vi "Mediaplayer play.vi"(0 "music":string(combo)="0", 2 "MediaPlayer":refnum<k7>(container), 3 "error in":errorcluster) -> (7 "error out":errorcluster)   [LabVIEW 2010]
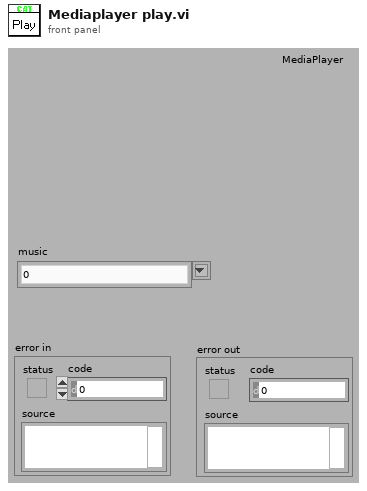
[diagram p1: front panel]
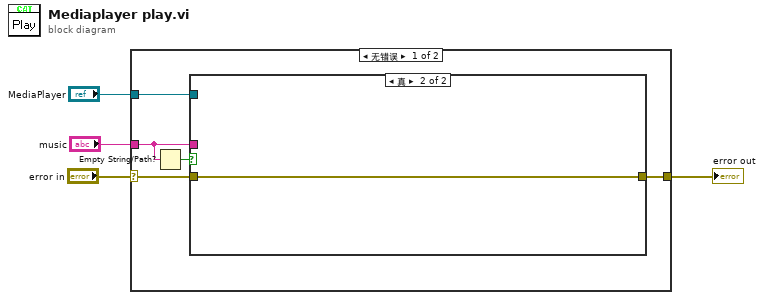
[diagram p0: block diagram]
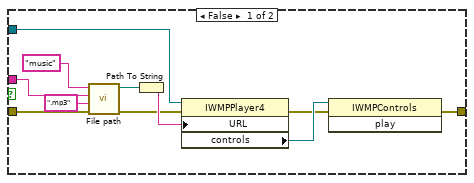
[diagram p2: hidden frame]
diagram:
  n1 = case shown="无错误" "error in" {
    selector: "error in" -> [w7 w22]
    tunnel: "music" -> [w5 _]
    tunnel: [w8 w22] -> w3
    tunnel: "MediaPlayer" -> [w9 _]
    frame No Error {
      n2 = Empty String/Path?(string/path=w5) -> (empty?=w6:bool)
      n3 = case shown="真" w6 {
        tunnel: w5 -> [w19 _]
        tunnel: w9 -> [w16 _]
        tunnel: [w13 w21] -> w8
        tunnel: w7 -> [w12 w21]
        frame False {
          n4 = call "File path.vi"("folder name"="music", "file name"=w19, "pattern"=".mp3", "error in (no error)"=w12) -> ("build path"=w11:path, "error out"=w17:errorcluster)  [unwired: 3 out]
          n5 = Path To String(path=w11) -> (string=w18:string)
          n6 = property class="IWMPPlayer4"(reference=w16, error in=w17, "URL"=w18) -> (error out=w14:errorcluster, "controls"=w15:refnum<k7>)  [unwired: 1 out]
          n7 = invoke class="IWMPControls" method="play"(reference=w15, error in=w14) -> (error out=w13:errorcluster)  [unwired: 1 in, 2 out]
        }
        frame True {
        }
      }
    }
    frame Error {
    }
  }
  "error out" <- w3
